vi "get_frequencies.vi"(8 "error in":errorcluster, 11 "Resonance Curve Data in":refnum<class "Resonance Curve Data.lvclass">) -> (0 "error out":errorcluster, 2 "Frequencies (Hz)":dbl[](array[numeric]), 3 "Resonance Curve Data out":refnum<class "Resonance Curve Data.lvclass">)   [LabVIEW 2020, in "Resonance Curve Data.lvclass"]
uses:
  Resonance Curve Data.lvclass
  Resonance Curve Data.lvclass/Resonance Curve Data.ctl
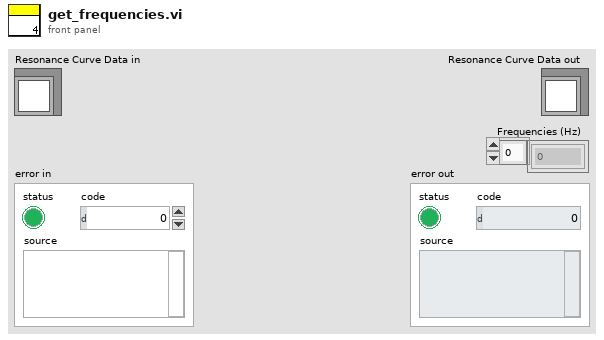
[diagram p1: front panel]
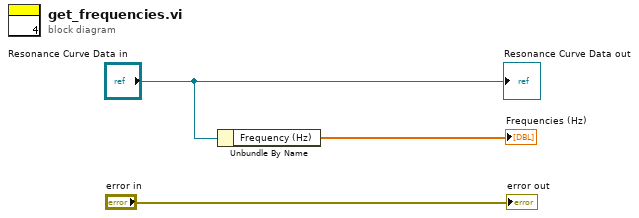
[diagram p0: block diagram]
diagram:
  n1 = Unbundle By Name("Resonance Curve Data in") -> ("Frequency (Hz)"=→"Frequencies (Hz)":dbl[])
  "Resonance Curve Data out" <- "Resonance Curve Data in"
  "error out" <- "error in"
